vi "obj_LuaVIEW Daemon Exchange.vi"(0 "method":T1, 5 "path in":path, 7 "static daemon reference {send path}":refnum<vi>, 11 "error reply in":errorcluster) -> (4 "available?":bool, 6 "path out":path, 8 "send occurrence":refnum<k4>, 10 "reply occurrence":refnum<k4>, 15 "error reply out":errorcluster)   [LabVIEW 2013]
doc: "This object serves to send messages to and receive replies from the Registry Daemon which manages the public function registry. The daemon is automatically launched when a path of a function VI to be registered is sent for the first time. Opening the function VI references via the daemon is required because LabVIEW inanely insists on and cannot be disuaded from automatically closing references when the top-level context in which references are opened terminates. Note that occurrences are used to have the sender notify the daemon and the replying deamon notify the sender. These must be set outside this VI after calling the respective send and reply methods. The reason for not including the setting of the occurrence in the methods is that this leads to superfluous context switches: in order to react to an occurrence, this VI must be called. To do so, no other caller may be using this VI. Thus, effecting a context switch while inside this VI would lead to a total of three context switches, the last two of which are scheduler instead of occurrence driven, thus causing more instead of less latency."
uses:
  typedefs/t_LuaVIEW Daemon Exchange Methods.ctl
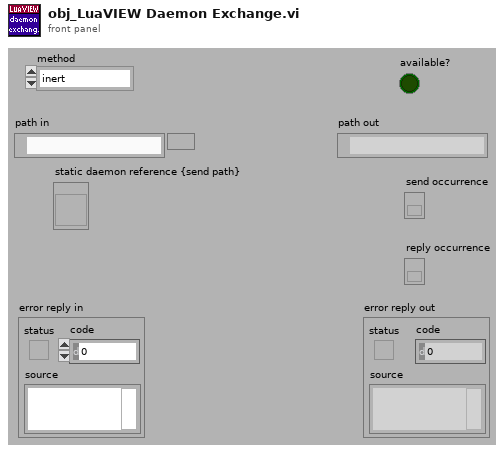
[diagram p1: front panel]
types:
  T1 = typedef "t_LuaVIEW Daemon Exchange Methods.ctl" = enum16{"inert", "send path", "send cleanup", "get sent", "reply", "get reply", "unset launched"}
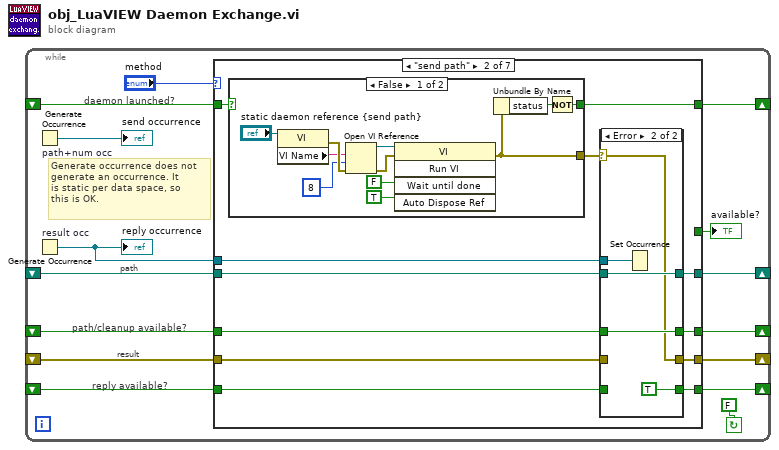
[diagram p0: block diagram]
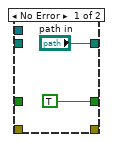
[diagram p3: hidden frame]
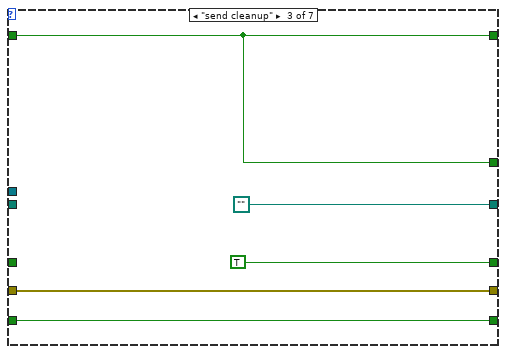
[diagram p5: hidden frame]
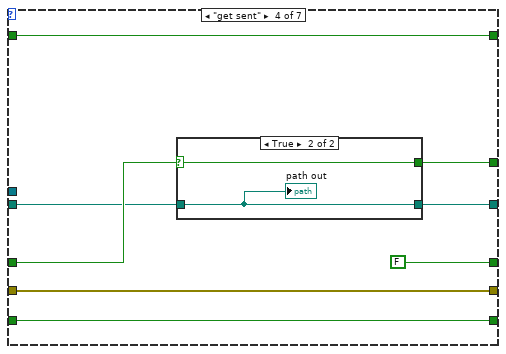
[diagram p6: hidden frame]
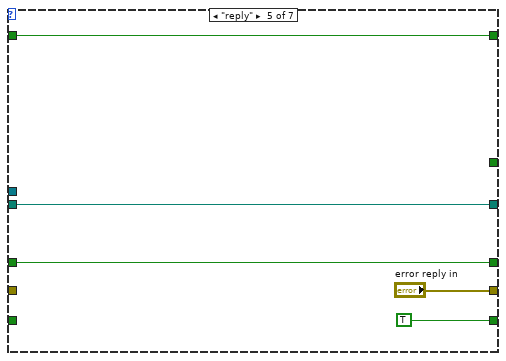
[diagram p8: hidden frame]
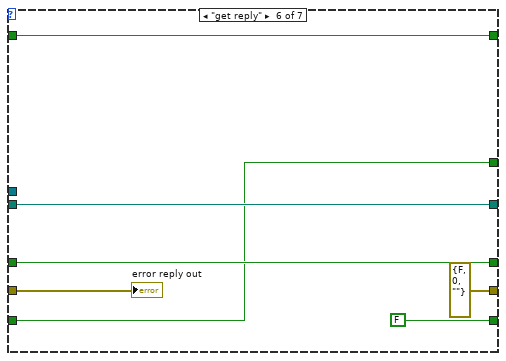
[diagram p9: hidden frame]
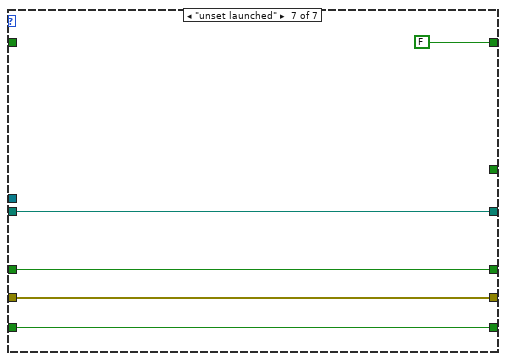
[diagram p10: hidden frame]
diagram:
  n1 = while {
    shift-right: [w10] -> _
    shift-left: _ -> [w13]
    shift-right: [w12] -> _
    shift-left: _ -> [w11]
    shift-right: [w8] -> _
    shift-left: _ -> [w9]
    shift-right: [w6] -> _
    shift-left: _ -> [w7]
    shift-right: [w2] -> _
    shift-left: _ -> [w3]
    stop <- FALSE continue-if-true
    # "Generate occurrence does not\ngenerate an occurrence. It\nis static per data space, so\nthis is OK."
    # "daemon launched?"
    # "path/cleanup available?"
    # "reply available?"
    # "result"
    # "path"
    n2 = Generate Occurrence "path+num occ"() -> (→"send occurrence":refnum<k4>)
    n3 = Generate Occurrence "result occ"() -> (w1:refnum<k4>)
    "reply occurrence" <- w1
    n4 = case shown="\"send path\"" "method" {
      tunnel: w13 -> [w19 w28 w55 w63 _ w75 w81]
      tunnel: w11 -> [w17 w24 _ w61 w73 w80 w83]
      tunnel: [w17 w31 TRUE FALSE w73 w80 w83] -> w12
      tunnel: [w19 w27 w55 w63 "error reply in" errorcluster {"status"=FALSE, "code"=0, "source"=""} w81] -> w10
      tunnel: [w18 w32 path "" w59 w72 w79 w85] -> w8
      tunnel: w9 -> [w18 w25 _ w58 w72 w79 w85]
      tunnel: w7 -> [w20 w23 w56 w64 _ w77 w82]
      tunnel: [w20 w22 w56 w64 TRUE FALSE w82] -> w6
      tunnel: [_ _ w52 w60 _ w77 _] -> w4
      tunnel: w3 -> [w16 w30 w52 w57 w69 w76 _]
      tunnel: [w16 w29 w52 w57 w69 w76 FALSE] -> w2
      tunnel: w1 -> [_ w21 _ _ _ _ _]
      frame "inert" {
      }
      frame "send path" {
        n5 = case shown="False" w30 {
          selector: w30 -> [_ w51]
          tunnel: [w46 w51] -> w29
          tunnel: [w44 _] -> w26
          frame False {
            n6 = property class="VI"(reference="static daemon reference {send path}") -> (error out=w50:errorcluster, "VI Name"=w41:string)  [unwired: 1 in, 1 out]
            n7 = Open VI Reference(vi path=w41, options=8, error in (no error)=w50) -> (vi reference=w47:refnum<vi>, error out=w43:errorcluster)  [unwired: 3 in]
            n8 = invoke class="VI" method="Run VI"(reference=w47, error in=w43, "Wait until done"=FALSE, "Auto Dispose Ref"=TRUE) -> (error out=w44:errorcluster)  [unwired: 1 in, 4 out]
            n9 = Unbundle By Name(w44) -> ("status"=w45:bool)
            n10 = Not(x=w45) -> (.not. x?=w46:bool)
          }
          frame True {
          }
        }
        n11 = case shown="Error" w26 {
          selector: w26 -> [_ w37]
          tunnel: ["path in" w39] -> w32
          tunnel: [TRUE w38] -> w31
          tunnel: w28 -> [_ _]
          tunnel: [_ w37] -> w27
          tunnel: w25 -> [_ w39]
          tunnel: w24 -> [_ w38]
          tunnel: w23 -> [_ _]
          tunnel: [_ TRUE] -> w22
          tunnel: w21 -> [_ w36]
          frame No Error {
          }
          frame Error {
            n12 = Set Occurrence(w36) -> ()
          }
        }
      }
      frame "send cleanup" {
      }
      frame "get sent" {
        n13 = case shown="True" w61 {
          selector: w61 -> [w66 w68]
          tunnel: [w66 w68] -> w60
          tunnel: [w65 w67] -> w59
          tunnel: w58 -> [w65 w67]
          frame False {
          }
          frame True {
            "path out" <- w67
          }
        }
      }
      frame "reply" {
      }
      frame "get reply" {
        "error reply out" <- w75
      }
      frame "unset launched" {
      }
    }
    "available?" <- w4
  }
